vi "shutter port lookup.vi"(1 "Shutter name":T1) -> (0 "Shutter Device and port":tag)   [LabVIEW 2016]
uses:
  Laser type.ctt
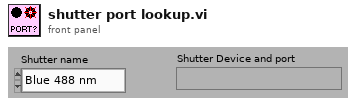
[diagram p1: front panel]
types:
  T1 = typedef "Laser type.ctt" = enum16{"Blue 488 nm", "Green 532 nm", "Red 635 nm", "IR 785"}
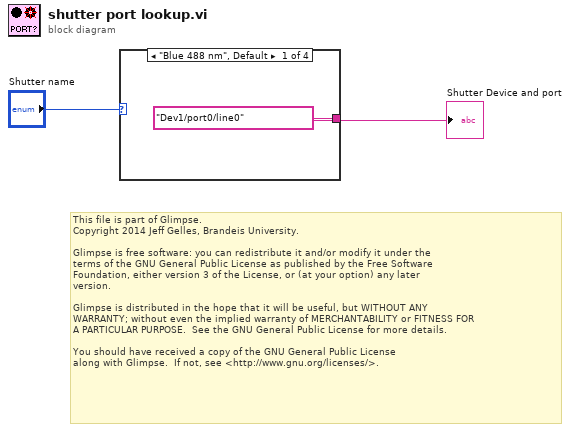
[diagram p0: block diagram]
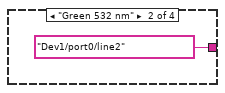
[diagram p2: hidden frame]
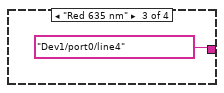
[diagram p3: hidden frame]
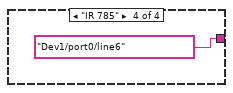
[diagram p4: hidden frame]
diagram:
  # "This file is part of Glimpse. \nCopyright 2014 Jeff Gelles, Brandeis University.    \n\nGlimpse is free software: you can redistribute it and/or modify it under the \nterms of the GNU General Public License as published by the Free Software \nFoundation, either version 3 of the License, or (at your option) any later \nversion.\n\nGlimpse is distributed in the hope that it will be useful, but WITHOUT ANY \nWARRANTY; without even the implied warranty of MERCHANTABILITY or FITNESS FOR \nA PARTICULAR PURPOSE.  See the GNU General Public License for more details.\n\nYou should have received a copy of the GNU General Public License\nalong with Glimpse.  If not, see <http://www.gnu.org/licenses/>."
  n1 = case shown="\"Blue 488 nm\", Default" "Shutter name" {
    tunnel: [tag "Dev1/port0/line0" ("lines") tag "Dev1/port0/line2" ("lines") tag "Dev1/port0/line4" ("lines") tag "Dev1/port0/line6" ("lines")] -> w2
    frame "Blue 488 nm", Default {
    }
    frame "Green 532 nm" {
    }
    frame "Red 635 nm" {
    }
    frame "IR 785" {
    }
  }
  "Shutter Device and port" <- w2
